vi "New LINX-PCA9685 PWM.vi"(8 "error in (no error)":errorcluster, 10 "I2C Slave Address (0x40)":u8=64 format="%.0x", 11 "I2C":refnum<class "LINX I2C.lvclass">) -> (0 "error out":errorcluster, 3 "LINX-PCA9865 PWM out":refnum<class "LINX-PCA9685 PWM.lvclass">)   [LabVIEW 2020, in "LINX-PCA9685 PWM.lvclass"]
uses:
  LINX-PCA9685 PWM.lvclass
  LINX I2C/LINX I2C.lvclass
  LINX-PCA9685 PWM.lvclass/LINX-PCA9685 PWM.ctl
  Write I2C Slave Address (0x40).vi
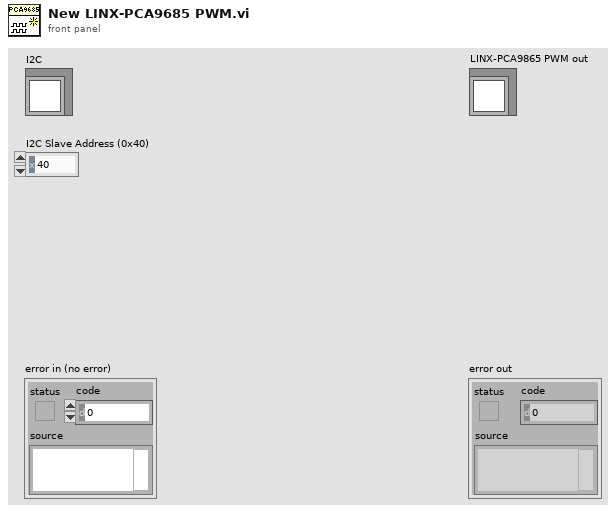
[diagram p1: front panel]
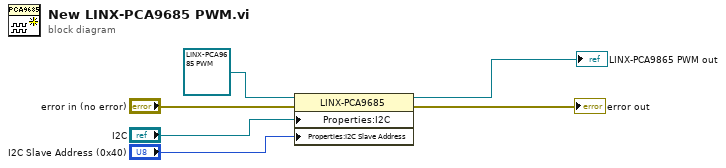
[diagram p0: block diagram]
diagram:
  n1 = property class="LINX-PCA9685"(reference=refnum<class "LINX-PCA9685 PWM.lvclass"> refnum ("LINX-PCA9865 PWM in"), error in="error in (no error)", "Properties:I2C"="I2C", "Properties:I2C Slave Address"="I2C Slave Address (0x40)") -> (reference out=→"LINX-PCA9865 PWM out":refnum<class "LINX-PCA9685 PWM.lvclass">, error out=→"error out":errorcluster)
